vi "isRunning.vi"(8 "error in (no error)":errorcluster, 11 "TaskController in":refnum<class "TaskController.lvclass">) -> (0 "error out":errorcluster, 2 "isRunning":bool, 3 "TaskController out":refnum<class "TaskController.lvclass">)   [LabVIEW 2023, in "TLC_Daemon.lvlib" / "TaskController.lvclass"]
doc: "is the task running?"
uses:
  TaskController.lvclass
  ITask/ITask.lvclass
  ITaskStopMechanism/ITaskStopMechanism.lvclass
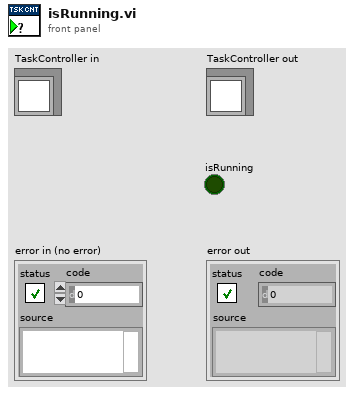
[diagram p1: front panel]
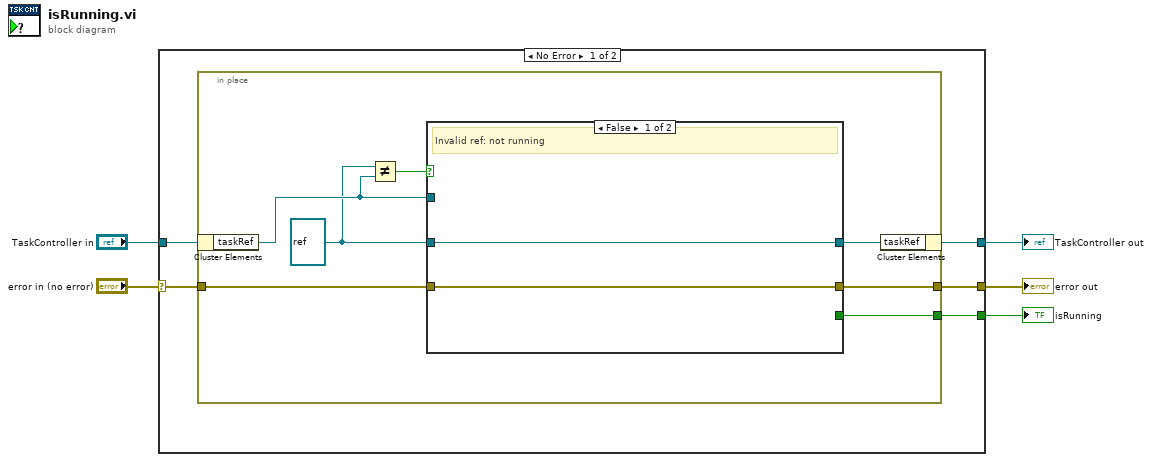
[diagram p0: block diagram]
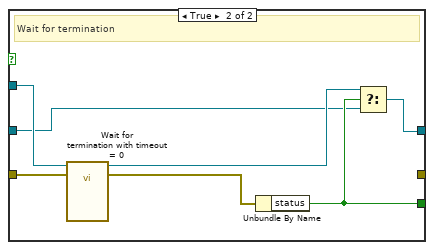
[diagram p2: hidden frame]
diagram:
  n1 = case shown="No Error" "error in (no error)" {
    selector: "error in (no error)" -> [w7 w28]
    tunnel: [w8 w28] -> w4
    tunnel: [w10 w27] -> w2
    tunnel: "TaskController in" -> [w9 w27]
    tunnel: [w6 _] -> w1
    frame No Error {
      n2 = in-place {
        in-place-border: w7 -> [w17]
        in-place-border: [w16] -> w8
        in-place-border: [w14] -> w6
        w11 = refnum<vi> refnum ("x")
        n3 = in-place-cluster #1(w9) -> ("taskRef"=w13:refnum<vi>)
        n4 = Not Equal?(x=w11, y=w13) -> (x != y?=w15:bool)
        n5 = case shown="False" w15 {
          tunnel: w17 -> [w19 w25]
          tunnel: w13 -> [_ w26]
          tunnel: [w19 _] -> w16
          tunnel: [_ w23] -> w14
          tunnel: [w18 w21] -> w12
          tunnel: w11 -> [w18 w20]
          frame False {
            # "Invalid ref: not running"
          }
          frame True {
            # "Wait for termination"
            n6 = call-by-ref "Wait for\ntermination with timeout = 0"(reference=w26, error in=w25) -> (reference out=w22:refnum<vi>, error out=w24:errorcluster)  [unwired: 10 in, 2 out]
            n7 = Unbundle By Name(w24) -> ("status"=w23:bool)
            n8 = Select(t=w22, s=w23, f=w20) -> (s? t:f=w21:refnum<vi>)
          }
        }
        n9 = in-place-cluster #1("taskRef"=w12) -> (w10:refnum<class "TaskController.lvclass">)
      }
    }
    frame Error {
    }
  }
  "error out" <- w4
  "TaskController out" <- w2
  "isRunning" <- w1
